vi "SumAroundPeak_IQ.vi"(7 "MaxIndex":i32, 11 "spectrum in":dbl[](array[numeric])) -> (0 "ZoomSpectrumNeg":dbl[](array[numeric]), 1 "Positive Max":dbl, 2 "Negative_Max":dbl, 3 "PosZoomSpect":dbl[](array[numeric]), 4 "ZoomSpectrumPos":dbl[](array[numeric]), 5 "NegZoomSpect":dbl[](array[numeric]))   [LabVIEW 2018]
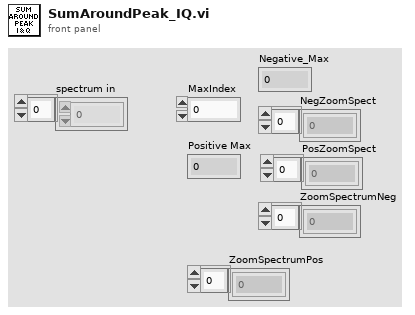
[diagram p1: front panel]
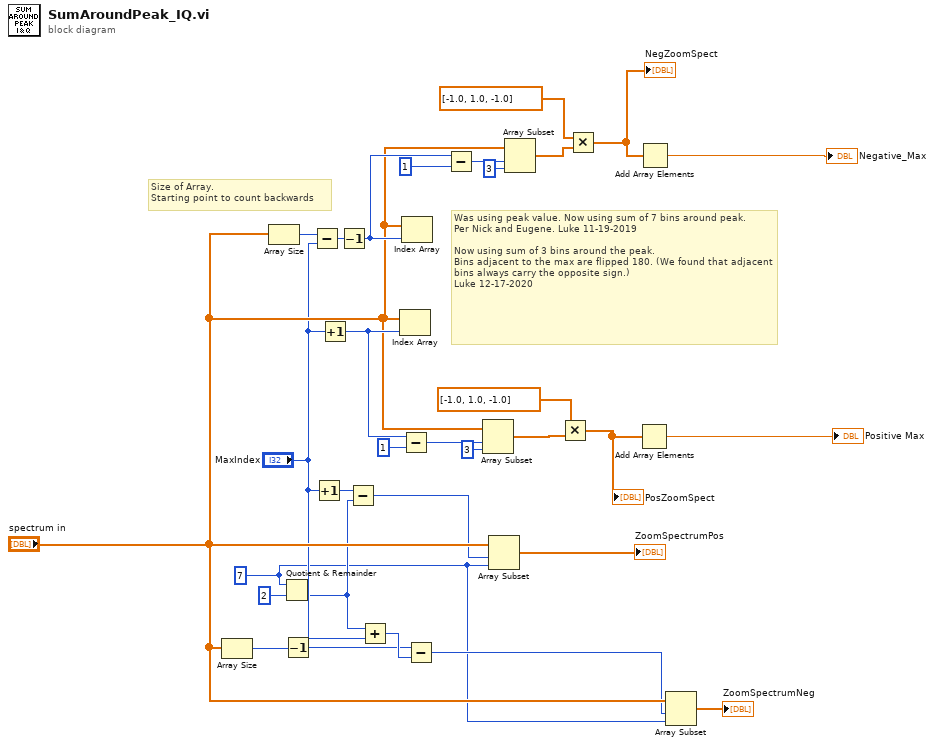
[diagram p0: block diagram]
diagram:
  w12 = 7 ("ZoomWidth")
  # "Size of Array.\nStarting point to count backwards"
  # "Was using peak value. Now using sum of 7 bins around peak.\nPer Nick and Eugene. Luke 11-19-2019\n\nNow using sum of 3 bins around the peak.\nBins adjacent to the max are flipped 180. (We found that adjacent bins always carry the opposite sign.)\nLuke 12-17-2020"
  n1 = Array Size(array="spectrum in") -> (size(s)=w18:i32)
  n2 = Array Size(array="spectrum in") -> (size(s)=w29:i32)
  n3 = Quotient & Remainder(x=w12, y=2) -> (floor(x/y)=w15:i32)  [unwired: 1 out]
  n4 = Decrement(x=w18) -> (x-1=w9:i32)
  n5 = Subtract(x=w29, y="MaxIndex") -> (x-y=w28:i32)
  n6 = Increment(x="MaxIndex") -> (x+1=w10:i32)
  n7 = Increment(x="MaxIndex") -> (x+1=w25:i32)
  n8 = Decrement(x=w28) -> (x-1=w20:i32)
  n9 = Subtract(x=w10, y=w15) -> (x-y=w17:i32)
  n10 = Add(x=w15, y="MaxIndex") -> (x+y=w14:i32)
  n11 = Index Array(array="spectrum in", index=w25) -> ()  [unwired: 1 out]
  n12 = Subtract(x=w25, y=1) -> (x-y=w26:i32)
  n13 = Index Array(array="spectrum in", index=w20) -> ()  [unwired: 1 out]
  n14 = Subtract(x=w9, y=w14) -> (x-y=w13:i32)
  n15 = Subtract(x=w20, y=1) -> (x-y=w22:i32)
  n16 = Array Subset(array="spectrum in", index=w26, length=3) -> (w5:dbl[])
  n17 = Array Subset(array="spectrum in", index=w17, length=w12) -> (→"ZoomSpectrumPos":dbl[])
  n18 = Array Subset(array="spectrum in", index=w22, length=3) -> (w8:dbl[])
  n19 = Multiply(x=dbl[] [-1.0, 1.0, -1.0], y=w5) -> (x*y=w3:dbl[])
  "PosZoomSpect" <- w3
  n20 = Multiply(x=dbl[] [-1.0, 1.0, -1.0], y=w8) -> (x*y=w7:dbl[])
  "NegZoomSpect" <- w7
  n21 = Add Array Elements(numeric array=w3) -> (sum=→"Positive Max":dbl)
  n22 = Add Array Elements(numeric array=w7) -> (sum=→"Negative_Max":dbl)
  n23 = Array Subset(array="spectrum in", index=w13, length=w12) -> (→"ZoomSpectrumNeg":dbl[])
